vi "update anott. position.vi"(8 "error in (no error)":errorcluster, 9 "Annotation No":i32, 10 "y axis min.":dbl, 11 "XYGraph in":refnum<vi>) -> (0 "error out":errorcluster, 3 "XYGraph out":refnum<vi>)   [LabVIEW 2014]
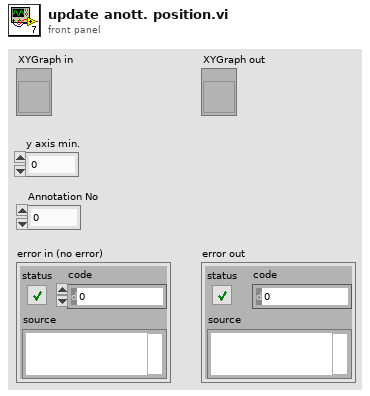
[diagram p1: front panel]
types:
  T1 = typedef "LVAnnotationListTypeDef.ctl" = cluster{"Name":string, "Color":u32, "Style":u8, "Point Style":u8, "Name Visible":bool, "Allow Drag":bool, "Annotation Mode":u32, "Plot":i32, "Index":i32, "Position":cluster{"X":dbl, "Y":dbl}, "X Scale":u32, "Y Scale":u32, "Show Arrow":bool, "Lock Name":bool, "Plot Area":i32, "Label Offset":cluster{"X":dbl, "Y":dbl}}[]
  T2 = cluster{"Name":string, "Color":u32, "Style":u8, "Point Style":u8, "Name Visible":bool, "Allow Drag":bool, "Annotation Mode":u32, "Plot":i32, "Index":i32, "Position":cluster{"X":dbl, "Y":dbl}, "X Scale":u32, "Y Scale":u32, "Show Arrow":bool, "Lock Name":bool, "Plot Area":i32, "Label Offset":cluster{"X":dbl, "Y":dbl}}
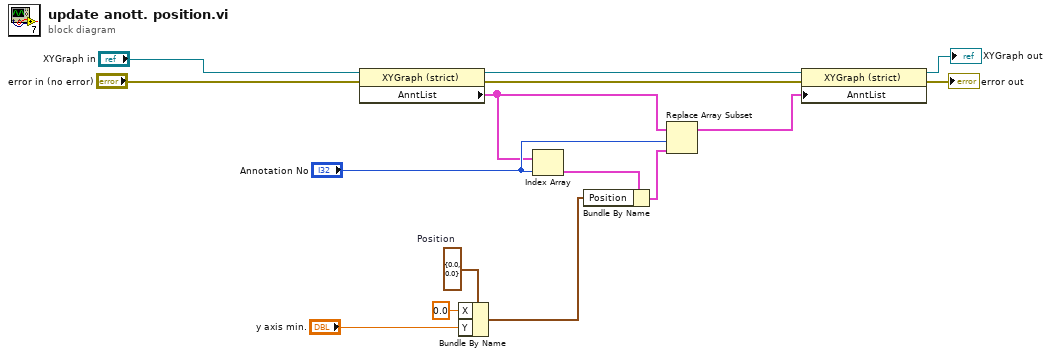
[diagram p0: block diagram]
diagram:
  w6 = cluster{"X":dbl, "Y":dbl} {"X"=0.0, "Y"=0.0}  # Position
  n1 = property class="XYGraph (strict)"(reference="XYGraph in", error in="error in (no error)") -> (reference out=w12:refnum<vi>, error out=w10:errorcluster, "AnntList"=w7:T1)
  n2 = Bundle By Name(cluster=w6, "X"=0.0, "Y"="y axis min.") -> (w4:cluster{"X":dbl, "Y":dbl})
  n3 = Index Array(array=w7, index="Annotation No") -> (element=w13:T2)
  n4 = Bundle By Name(cluster=w13, "Position"=w4) -> (w14:T2)
  n5 = Replace Array Subset "Replace Array Subset"(array=w7, new element=w14, index="Annotation No") -> (w8:T1)
  n6 = property class="XYGraph (strict)"(reference=w12, error in=w10, "AnntList"=w8) -> (reference out=→"XYGraph out":refnum<vi>, error out=→"error out":errorcluster)
